vi "AC DC Coupling.vi"(0 "voltage waveforms in":waveform(dbl)[](array[waveform]), 5 "current waveforms in":waveform(dbl)[](array[waveform]), 7 "coupling":enum16{"DC coupling", "AC coupling"}(ring), 9 "system info in":refnum<class "EP System Info.lvclass">, 11 "error in (no error)":errorcluster) -> (4 "voltage waveforms out":waveform(dbl)[](array[waveform]), 6 "current waveforms out":waveform(dbl)[](array[waveform]), 10 "system info out":refnum<class "EP System Info.lvclass">, 15 "error out":errorcluster)   [LabVIEW 2014, in "NI_EP_Power Quality.lvlib"]
doc: "Eliminates the DC component of voltage waveforms, current waveforms, or waveforms that contain both voltage and current.\n\nThis VI supports measuring single-line and multiple-line systems."
uses:
  <vilib>/addons/Electrical Power/PQ/NI_EP_Power Quality.lvlib
  <vilib>/addons/Electrical Power/PQ/Common/Classes/System Info/EP System Info.lvclass
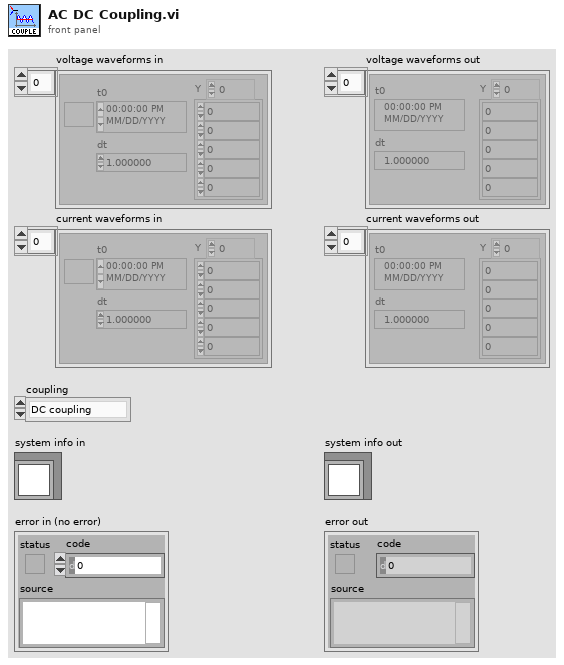
[diagram p1: front panel]
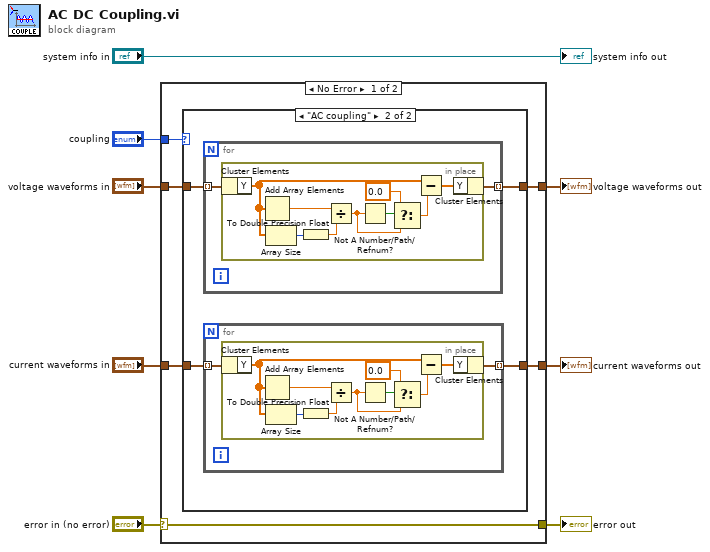
[diagram p0: block diagram]
diagram:
  n1 = case shown="No Error" "error in (no error)" {
    selector: "error in (no error)" -> [w9 w45]
    tunnel: "voltage waveforms in" -> [w14 w44]
    tunnel: [w13 w44] -> w6
    tunnel: "current waveforms in" -> [w12 w43]
    tunnel: [w11 w43] -> w5
    tunnel: "coupling" -> [w10 _]
    tunnel: [w9 w45] -> w2
    frame No Error {
      n2 = case shown="\"AC coupling\"" w10 {
        tunnel: w14 -> [w16 w20]
        tunnel: [w16 w19] -> w13
        tunnel: w12 -> [w15 w18]
        tunnel: [w15 w17] -> w11
        frame "DC coupling", Default {
        }
        frame "AC coupling" {
          n3 = for {
            tunnel: w20 -> [w33] mode=indexing
            tunnel: [w32] -> w19 mode=indexing
            n4 = in-place {
              n5 = in-place-cluster #1(w33) -> ("Y"=w36:dbl[])
              n6 = Add Array Elements(numeric array=w36) -> (sum=w41:dbl)
              n7 = Array Size(array=w36) -> (size(s)=w40:i32)
              n8 = To Double Precision Float(number=w40) -> (double precision float=w39:dbl)
              n9 = Divide(x=w41, y=w39) -> (x/y=w38:dbl)
              n10 = Not A Number/Path/Refnum?(number/path/refnum=w38) -> (NaN/Path/Refnum?=w42:bool)
              n11 = Select(t=0.0, s=w42, f=w38) -> (s? t:f=w34:dbl)
              n12 = Subtract(x=w36, y=w34) -> (x-y=w35:dbl[])
              n13 = in-place-cluster #1("Y"=w35) -> (w32:waveform(dbl))
            }
          }
          n14 = for {
            tunnel: w18 -> [w22] mode=indexing
            tunnel: [w21] -> w17 mode=indexing
            n15 = in-place {
              n16 = in-place-cluster #2(w22) -> ("Y"=w25:dbl[])
              n17 = Add Array Elements(numeric array=w25) -> (sum=w30:dbl)
              n18 = Array Size(array=w25) -> (size(s)=w29:i32)
              n19 = To Double Precision Float(number=w29) -> (double precision float=w28:dbl)
              n20 = Divide(x=w30, y=w28) -> (x/y=w27:dbl)
              n21 = Not A Number/Path/Refnum?(number/path/refnum=w27) -> (NaN/Path/Refnum?=w31:bool)
              n22 = Select(t=0.0, s=w31, f=w27) -> (s? t:f=w23:dbl)
              n23 = Subtract(x=w25, y=w23) -> (x-y=w24:dbl[])
              n24 = in-place-cluster #2("Y"=w24) -> (w21:waveform(dbl))
            }
          }
        }
      }
    }
    frame Error {
    }
  }
  "voltage waveforms out" <- w6
  "error out" <- w2
  "current waveforms out" <- w5
  "system info out" <- "system info in"
